vi "VI Tree.vi"   [LabVIEW 2012, in "Phidget Resistance Input.lvlib"]
doc: "${ResistanceInput:VITreeHeader}"
uses:
  <instrlib>/Phidgets/Phidget Resistance Input/Phidget Resistance Input.lvlib
  <instrlib>/Phidgets/Phidget Resistance Input/Public/ResistanceInputStart.vi
  <instrlib>/Phidgets/Phidget Resistance Input/Public/ResistanceInputOpen.vi
  <instrlib>/Phidgets/Phidget Resistance Input/Public/ResistanceInputClose.vi
panel:
  # "(c) 2015 Phidgets Inc..  ALL RIGHTS RESERVED."
  # "SEE DIAGRAM\nFOR VI TREE."
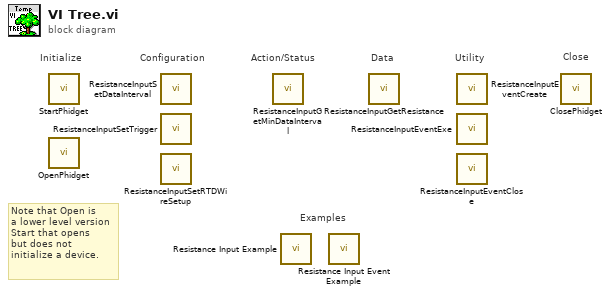
[diagram p0: block diagram]
diagram:
  # "Note that Open is\na lower level version\nStart that opens\nbut does not \ninitialize a device."
  # "Examples"
  # "Configuration"
  # "Utility"
  # "Data"
  # "Action/Status"
  # "Close"
  # "Initialize"
  n1 = call-poly <instrlib>:"StartPhidget.vi"() -> ()  [unwired: 12 in, 4 out]
  n2 = call-poly <instrlib>:"OpenPhidget.vi"() -> ()  [unwired: 8 in, 4 out]
  n3 = call <instrlib>:"ResistanceInputSetDataInterval.vi"() -> ()  [unwired: 9 in, 2 out]
  n4 = call <instrlib>:"ResistanceInputSetTrigger.vi"() -> ()  [unwired: 9 in, 2 out]
  n5 = call <instrlib>:"ResistanceInputSetRTDWireSetup.vi"() -> ()  [unwired: 9 in, 2 out]
  n6 = call <instrlib>:"ResistanceInputGetMinDataInterval.vi"() -> ()  [unwired: 8 in, 3 out]
  n7 = call <instrlib>:"Resistance Input Example.vi"() -> ()  [unwired: 12 in]
  n8 = call <instrlib>:"Resistance Input Event Example.vi"() -> ()  [unwired: 12 in]
  n9 = call <instrlib>:"ResistanceInputGetResistance.vi"() -> ()  [unwired: 8 in, 3 out]
  n10 = call <instrlib>:"ResistanceInputEventCreate.vi"() -> ()  [unwired: 9 in, 3 out]
  n11 = call <instrlib>:"ResistanceInputEventExe.vi"() -> ()  [unwired: 6 in, 6 out]
  n12 = call <instrlib>:"ResistanceInputEventClose.vi"() -> ()  [unwired: 10 in, 2 out]
  n13 = call-poly <instrlib>:"ClosePhidget.vi"() -> ()  [unwired: 11 in, 1 out]
